vi "Low Power Mode.vi"(0 "GEA2 Reference In":refnum<k24>, 5 "Action":enum16{"Enter", "Exit"}(ring), 11 "Error In":errorcluster) -> (4 "GEA2 Reference Out":refnum<k24>, 6 "Pass/Fail?":bool, 8 "Report Text":string, 15 "Error Out":errorcluster)   [LabVIEW 2018, in "TL27.lvlib"]
doc: "Use this VI to enter or exit low power mode."
uses:
  Projects/TL27.lvlib
  D:/Common/LabVIEW GEA2 Toolkit/source/GEA3 DLL Source/GeaCommunication.dll
  Common/LabVIEW GEA2 Toolkit/source/GEA3 DLL Source/GeaCommunication.dll
  Common/LabVIEW GEA2 Toolkit/GEA3/type defs/Source_Destination.ctl
  Common/LabVIEW GEA2 Toolkit/GEA3/type defs/ERD Read Data In.ctl
  Common/LabVIEW GEA2 Toolkit/GEA3/type defs/Data Type.ctl
  Common/LabVIEW GEA2 Toolkit/GEA3/type defs/ERD Write Data In.ctl
  C:/Users/iallatyp/Desktop/New folder/GEA3/library/GEA2_Toolkit.lvlib
panel:
  in  "Standalone?":bool
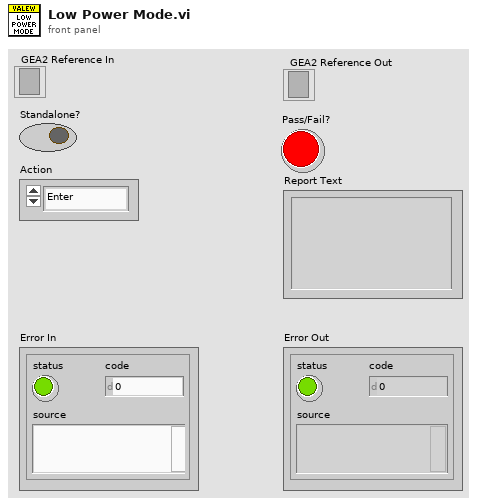
[diagram p1: front panel]
types:
  T1 = typedef "GEA2_Toolkit.lvlib/ERD Read Data In.ctl" = cluster{"ERD Number":u16, "Data Type":T2}
  T2 = typedef "GEA2_Toolkit.lvlib/Data Type.ctl" = enum16{"string", "boolean", "uint8_t", "uint16_t", "uint32_t", "uint64_t", "int8_t", "int16_t", "int32_t", "int64_t"}
  T3 = typedef "GEA2_Toolkit.lvlib/Source_Destination.ctl" = cluster{"Source":u8, "Destination":u8}
  T4 = typedef "GEA2_Toolkit.lvlib/ERD Write Data In.ctl" = cluster{"ERD Number":u16, "Data Type":T2, "Data":string}
  T5 = typedef "GEA2_Toolkit.lvlib/ERD Read Data Out.ctl" = cluster{"ERD Number":u16, "Data":string}
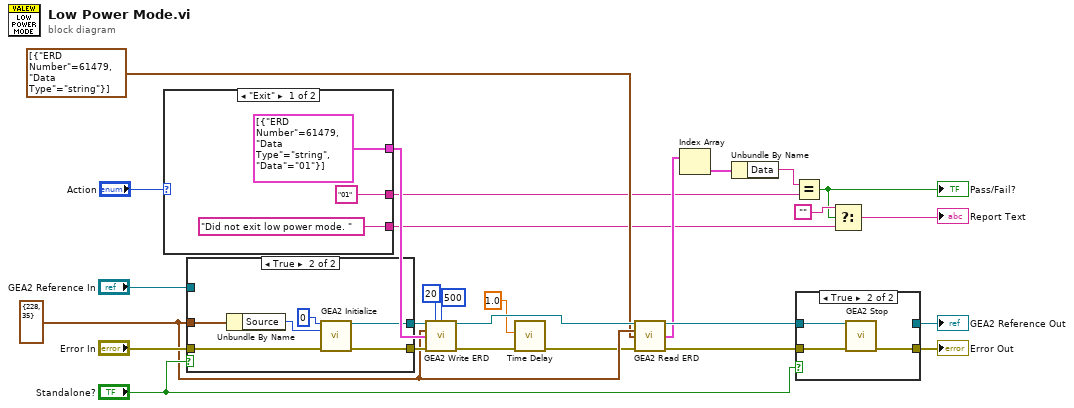
[diagram p0: block diagram]
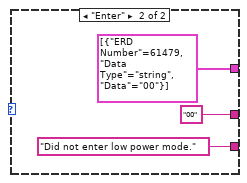
[diagram p2: hidden frame]
diagram:
  w18 = T3 {"Source"=228, "Destination"=35} ("GEA Inputs")
  n1 = case shown="\"Exit\"" "Action" {
    tunnel: [T4[] [{"ERD Number"=61479, "Data Type"=enum."string", "Data"="01"}] ("Write ERD List") T4[] [{"ERD Number"=61479, "Data Type"=enum."string", "Data"="00"}] ("Write ERD List")] -> w20
    tunnel: ["01" ("y") "00" ("y")] -> w7
    tunnel: ["Did not exit low power mode. " ("f") "Did not enter low power mode." ("f")] -> w6
    frame "Exit" {
    }
    frame "Enter" {
    }
  }
  n2 = case shown="True" "Standalone?" {
    tunnel: "Error In" -> [w34 w41]
    tunnel: [w34 w40] -> w21
    tunnel: "GEA2 Reference In" -> [w35 _]
    tunnel: [w35 w39] -> w27
    tunnel: w18 -> [_ w37]
    frame False {
    }
    frame True {
      n3 = Unbundle By Name(w37) -> ("Source"=w38:u8)
      n4 = call "GEA2 Initialize.vi"("Board Index"=0, "Source Address"=w38, "error in"=w41) -> ("GEA2 Reference Out"=w39:refnum<k24>, "error out"=w40:errorcluster)  [unwired: 10 in, 1 out]
    }
  }
  n5 = call "GEA2 Write ERD.vi"("GEA2 Reference In"=w27, "# of Tries"=u8 20, "Read Timeout (ms)"=u32 500, "GEA Inputs"=w18, "Write ERD List"=w20, "Error In"=w21) -> ("GEA2 Reference Out"=w19:refnum<k24>, "Error Out"=w2:errorcluster)  [unwired: 7 in, 1 out]
  n6 = call "Time Delay"("error in (no error)"=w2, "Delay Time (s)"=1.0) -> ("error out"=w1:errorcluster)  [unwired: 9 in]
  n7 = call "GEA2 Read ERD.vi"("GEA2 Reference In"=w19, "GEA Inputs"=w18, "Read ERD List"=T1[] [{"ERD Number"=61479, "Data Type"=enum."string"}], "Error In"=w1) -> ("GEA2 Reference Out"=w16:refnum<k24>, "ERD Data Out"=w12:T5[], "Error Out"=w15:errorcluster)  [unwired: 8 in, 1 out]
  n8 = Index Array(array=w12) -> (element=w11:T5)  [unwired: 1 in]
  n9 = Unbundle By Name(w11) -> ("Data"=w10:string)
  n10 = Equal?(x=w10, y=w7) -> (x = y?=w9:bool)
  "Pass/Fail?" <- w9
  n11 = case shown="True" "Standalone?" {
    tunnel: w15 -> [w43 w46]
    tunnel: [w43 w45] -> w26
    tunnel: [w42 _] -> w25
    tunnel: w16 -> [w42 w44]
    frame False {
    }
    frame True {
      n12 = call "GEA2 Stop.vi"("GEA2 Reference In"=w44, "Error In"=w46) -> ("Error Out"=w45:errorcluster)  [unwired: 13 in]
    }
  }
  "Error Out" <- w26
  "GEA2 Reference Out" <- w25
  n13 = Select(t="", s=w9, f=w6) -> (s? t:f=→"Report Text":string)
